vi "Write 1D Array of U32.vi"(7 "count (-1: all)":i64=-1 format="%d elements", 8 "error in (no error)":errorcluster, 9 "offset (0)":u64 format="%d bytes", 10 "buffer in":u32[](array[numeric]), 11 "Buffer in":refnum<class "Memory Buffer.lvclass">) -> (0 "error out":errorcluster, 1 "offset out":u64 format="%d bytes", 2 "buffer out":u32[](array[numeric]), 3 "Buffer out":refnum<class "Memory Buffer.lvclass">)   [LabVIEW 2017, in "Data Sharing Framework Engine.lvlib" / "Memory Buffer.lvclass"]
uses:
  Memory Buffer.lvclass
  C:/Program Files (x86)/National Instruments/LabVIEW 2017/vi.lib/National Instruments/Memory Manager/Classes/Pointer/Memory.Pointer.lvclass
  <vilib>/National Instruments/Memory Manager/Classes/Pointer/Memory.Pointer.lvclass/Memory.Pointer.ctl
  <vilib>/National Instruments/Memory Manager/Classes/Pointer/Memory.Pointer.Write.1D.U32.vi
  <vilib>/National Instruments/Memory Manager/Classes/Pointer/Memory.Pointer.Write.No Check.1D.U32.vi
  <vilib>/National Instruments/Memory Manager/Classes/Pointer/Memory.Pointer.Parameter Check.Null Pointer.vi
  <vilib>/National Instruments/Memory Manager/Classes/Pointer/Memory.Pointer.Parameter Check.Subset.Power of 2.vi
  <vilib>/National Instruments/Memory Manager/Classes/Pointer/Memory.Pointer.Get Address.vi
  <vilib>/National Instruments/Memory Manager/Classes/Pointer/Memory.Pointer.Errors.vi
  <vilib>/National Instruments/Memory Manager/Classes/Pointer/Memory.Pointer.Errors.Null Pointer.vi
  <vilib>/National Instruments/Memory Manager/Classes/Pointer/Memory.Pointer.Errors.Out of Bounds.vi
  <vilib>/National Instruments/Memory Manager/Classes/Pointer/Memory.Pointer.Get Size.vi
  <vilib>/National Instruments/Memory Manager/Classes/Pointer/Memory.Pointer.Count to Size.Power of 2.vi
  <vilib>/National Instruments/Memory Manager/Classes/Pointer/Memory.Pointer.Errors.Create Error.vi
  <vilib>/NI/Static Error Handling/VIs/Static Error Handling.Source Buffer.Write.String.vi
  <vilib>/National Instruments/Memory Manager/Classes/Pointer/Memory.Pointer.Errors.Write Pointer Size.vi
  <vilib>/NI/Static Error Handling/VIs/Static Error Handling.Source Buffer.Write.Numeric.Scalar.Base10.vi
  <vilib>/NI/Static Error Handling/VIs/Static Error Handling.Source Buffer.Write.Numeric.Scalar.Base10 (U64).vi
  <vilib>/NI/Static Error Handling/VIs/Static Error Handling.Error Cluster Constant.vi
  <vilib>/NI/Static Error Handling/VIs/Static Error Handling.Error Cluster Constant (512B).vi
  <vilib>/NI/Static Error Handling/VIs/Static Error Handling.Parameters.Status.Set.vi
  <vilib>/NI/Static Error Handling/VIs/Static Error Handling.Parameters.Code.Set.vi
  <vilib>/NI/Static Error Handling/VIs/Static Error Handling.Parameters.VI Source.Set.vi
  <vilib>/National Instruments/Memory Manager/Constants/Memory.Constants.vi
  <vilib>/National Instruments/Memory Manager/Constants/Memory.Constants.Library Name.vi
  <vilib>/National Instruments/Memory Manager/Classes/Pointer/Memory.Pointer.Errors.Get Info.vi
  <vilib>/National Instruments/Memory Manager/Classes/Pointer/Memory.Pointer.lvclass
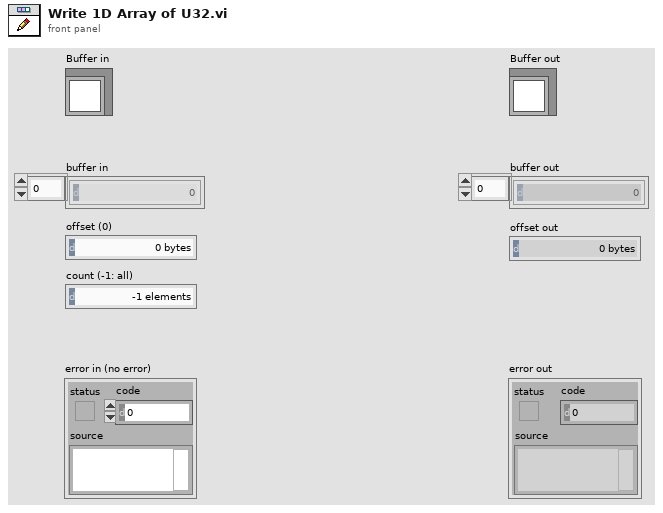
[diagram p1: front panel]
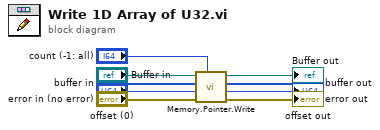
[diagram p0: block diagram]
diagram:
  n1 = call-poly <vilib>:"Memory.Pointer.Write.vi"("count (-1: all)"="count (-1: all)", "error in (no error)"="error in (no error)", "offset (0)"="offset (0)", "buffer in"="buffer in", "Pointer in"="Buffer in") -> ("error out"=→"error out":errorcluster, "offset out"=→"offset out":u64, "buffer out"=→"buffer out":u32[], "Pointer out"=→"Buffer out":refnum<class "Memory Buffer.lvclass">)  [unwired: 3 in]
